vi "未命名 1.vi"() -> ()   [LabVIEW 2018]
panel:
  out "A=B":bool
  out "A<B":bool
  out "A>B":bool
  out "SUM":dbl
  in  "B":dbl
  in  "A":dbl
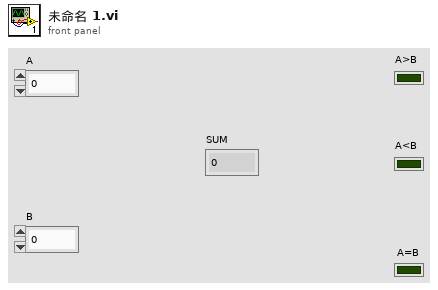
[diagram p1: front panel]
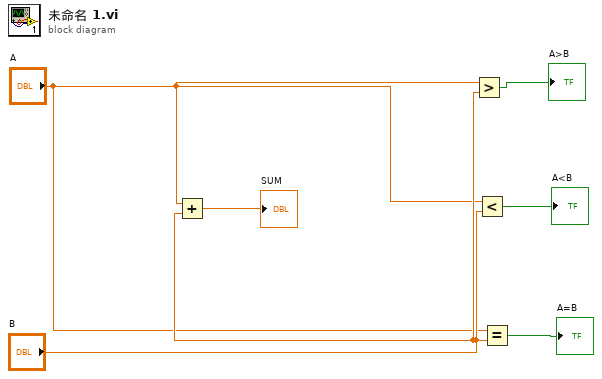
[diagram p0: block diagram]
diagram:
  n1 = Add(x="A", y="B") -> (x+y=→"SUM":dbl)
  n2 = Greater?(x="A", y="B") -> (0:→"A>B":bool)
  n3 = Less?(x="A", y="B") -> (x < y?=→"A<B":bool)
  n4 = Equal?(x="A", y="B") -> (x = y?=→"A=B":bool)
